vi "takeaveragebrightness.vi"(8 "Error In":errorcluster, 10 "Exposure (us)":u32, 11 "TLCamera reference in":refnum<k24>) -> (0 "Error Out":errorcluster, 2 "brightness":dbl, 3 "TLCamera reference out":refnum<k24>)   [LabVIEW 2019]
uses:
  C:/Users/jleeman/git_repos/CAxis_Machine/C-Axis LabView Controller/Library_X64/Thorlabs.TSI.TLCameraInterfaces.dll
  Library_X64/Thorlabs.TSI.TLCameraInterfaces.dll
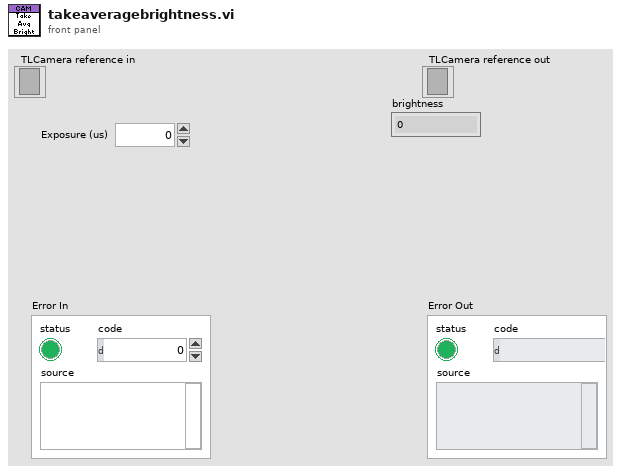
[diagram p1: front panel]
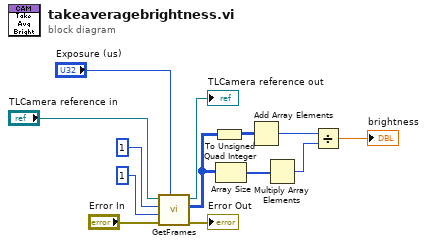
[diagram p0: block diagram]
diagram:
  n1 = call "GetFrames.vi"("ExposureTime_us"="Exposure (us)", "Error In"="Error In", "FramesPerTrigger"=u32 1, "Gain"=u32 1, "TLCamera reference in"="TLCamera reference in") -> ("Error Out"=→"Error Out":errorcluster, "Array"=w1:u16[][], "TLCamera reference out"=→"TLCamera reference out":refnum<k24>)  [unwired: 4 in]
  n2 = To Unsigned Quad Integer(1:w1) -> (0:w2:u64[][])
  n3 = Array Size(array=w1) -> (size(s)=w10:i32[])
  n4 = Add Array Elements(numeric array=w2) -> (sum=w11:u64)
  n5 = Multiply Array Elements(1:w10) -> (0:w9:i32)
  n6 = Divide(x=w11, y=w9) -> (x/y=→"brightness":dbl)
